vi "endsem.vi"() -> ()   [LabVIEW 2014]
uses:
  <vilib>/Analysis/NI_AALBase.lvlib
panel:
  out "XY Graph 2":cluster{dbl[], dbl[]}(graph)
  out "output cluster":cluster{dbl[], dbl[]}
  in  "standard deviation":dbl=1.0000000000000002 format="%0.2f"
  out "XY Graph":cdb[](graph)
  out "Array":i32[](array[numeric])
  in  "Numeric":i32
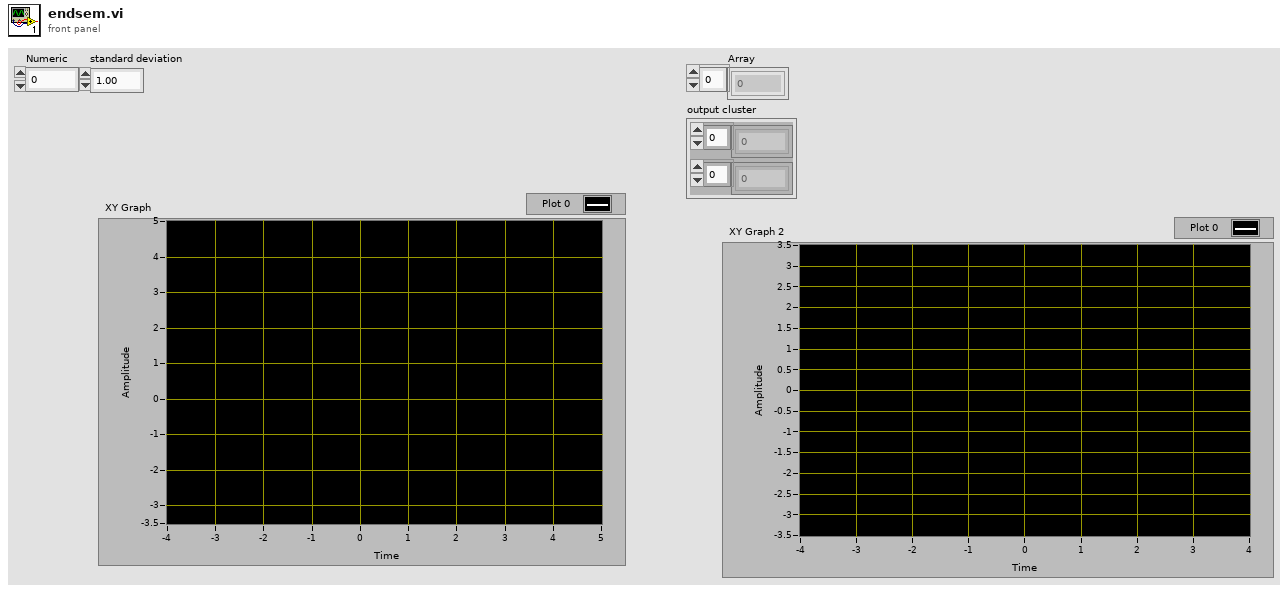
[diagram p1: front panel]
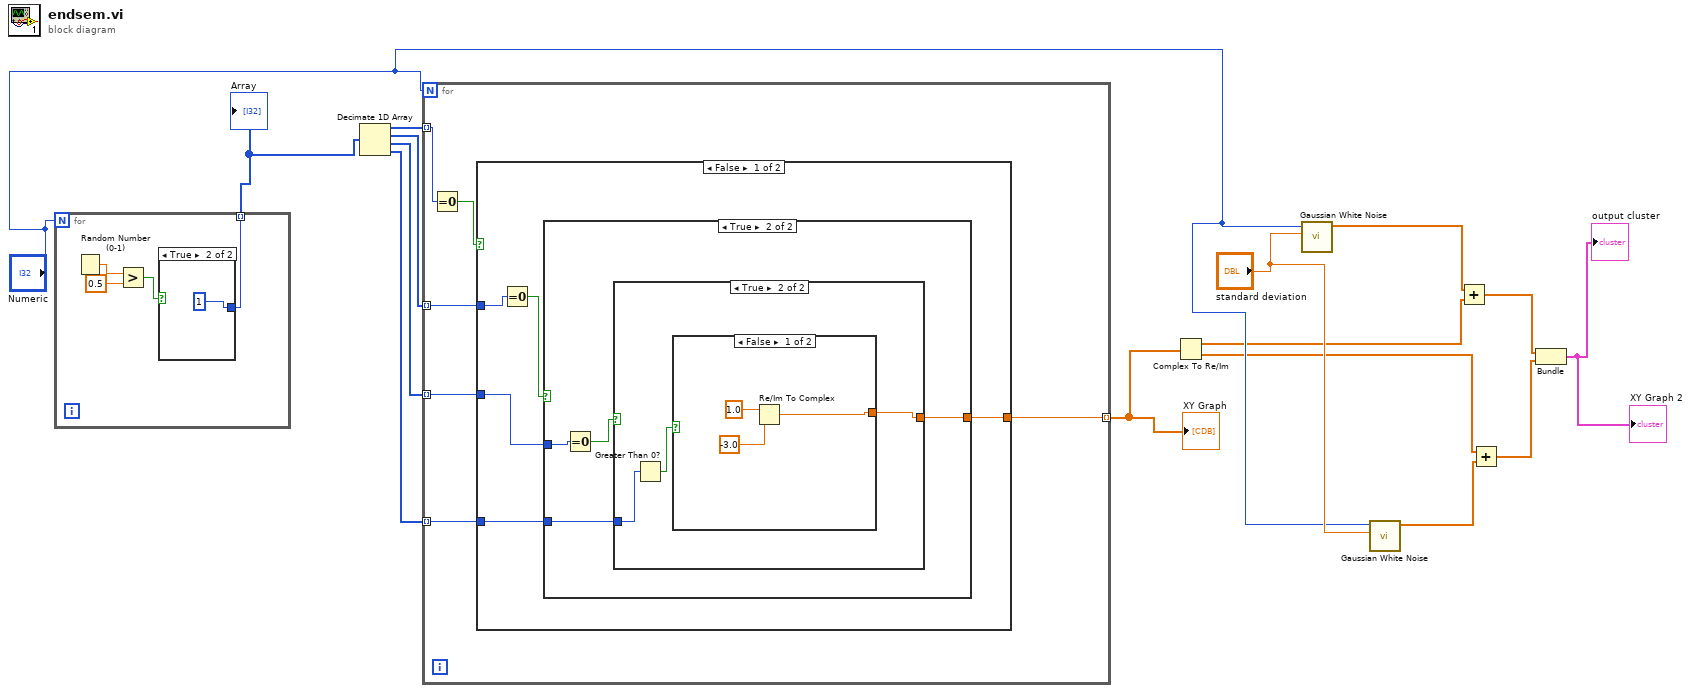
[diagram p0: block diagram]
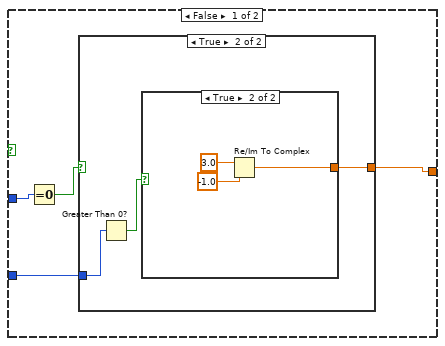
[diagram p2: hidden frame]
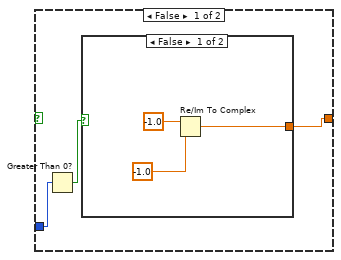
[diagram p3: hidden frame]
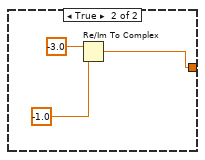
[diagram p4: hidden frame]
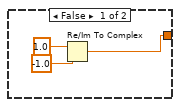
[diagram p5: hidden frame]
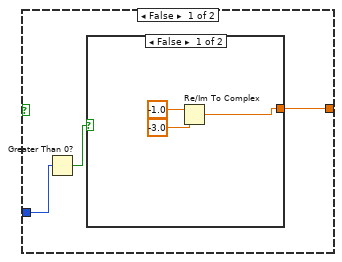
[diagram p6: hidden frame]
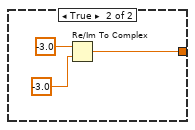
[diagram p7: hidden frame]
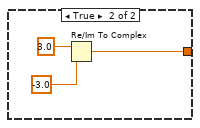
[diagram p8: hidden frame]
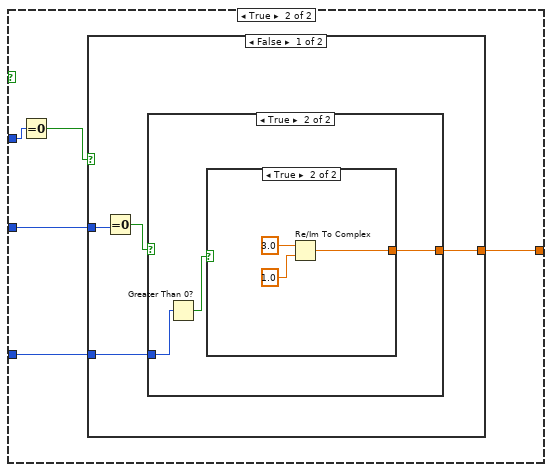
[diagram p9: hidden frame]
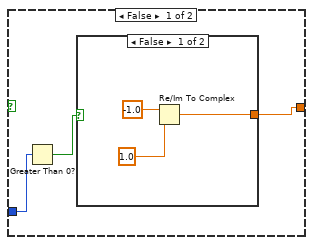
[diagram p10: hidden frame]
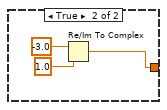
[diagram p11: hidden frame]
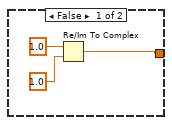
[diagram p12: hidden frame]
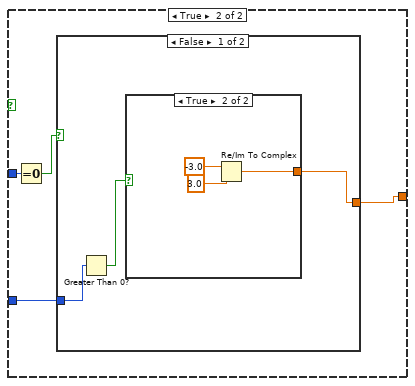
[diagram p13: hidden frame]
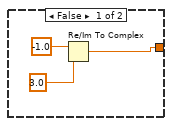
[diagram p14: hidden frame]
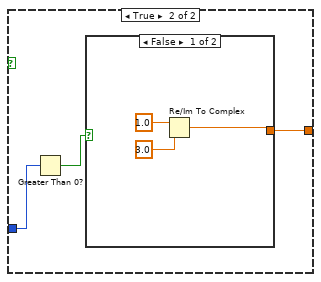
[diagram p15: hidden frame]
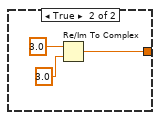
[diagram p16: hidden frame]
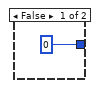
[diagram p17: hidden frame]
diagram:
  n1 = for {
    N: "Numeric" -> [_]
    tunnel: [w16] -> w15 mode=indexing
    n2 = Random Number (0-1)() -> (number: 0 to 1=w19:dbl)
    n3 = Greater?(x=w19, y=0.5) -> (0:w17:bool)
    n4 = case shown="True" w17 {
      tunnel: [0 1] -> w16
      frame False {
      }
      frame True {
      }
    }
  }
  "Array" <- w15
  n5 = Decimate 1D Array(w15) -> (w14:i32[], w13:i32[], w12:i32[], w11:i32[])
  n6 = for {
    N: "Numeric" -> [_]
    tunnel: w14 -> [w27] mode=indexing
    tunnel: w13 -> [w25] mode=indexing
    tunnel: w12 -> [w24] mode=indexing
    tunnel: w11 -> [w23] mode=indexing
    tunnel: [w22] -> w10 mode=indexing
    n7 = Equal To 0?(x=w27) -> (x = 0?=w26:bool)
    n8 = case shown="False" w26 {
      tunnel: w25 -> [w32 w81]
      tunnel: w24 -> [w30 w79]
      tunnel: w23 -> [w29 w78]
      tunnel: [w28 w77] -> w22
      frame False {
        n9 = Equal To 0?(x=w32) -> (x = 0?=w31:bool)
        n10 = case shown="True" w31 {
          tunnel: w30 -> [w36 w58]
          tunnel: w29 -> [w34 w56]
          tunnel: [w33 w55] -> w28
          frame False {
            n11 = Equal To 0?(x=w36) -> (x = 0?=w35:bool)
            n12 = case shown="True" w35 {
              tunnel: w34 -> [w39 w48]
              tunnel: [w37 w46] -> w33
              frame False {
                n13 = Greater Than 0?(x=w39) -> (x > 0?=w38:bool)
                n14 = case shown="False" w38 {
                  tunnel: [w40 w43] -> w37
                  frame False {
                    n15 = Re/Im To Complex(1:-1.0 ("y"), 2:-1.0 ("x")) -> (0:w40:cdb)
                  }
                  frame True {
                    n16 = Re/Im To Complex(1:-1.0 ("y"), 2:-3.0 ("x")) -> (0:w43:cdb)
                  }
                }
              }
              frame True {
                n17 = Greater Than 0?(x=w48) -> (x > 0?=w47:bool)
                n18 = case shown="True" w47 {
                  tunnel: [w49 w52] -> w46
                  frame False {
                    n19 = Re/Im To Complex(1:-1.0 ("y"), 2:1.0 ("x")) -> (0:w49:cdb)
                  }
                  frame True {
                    n20 = Re/Im To Complex(1:-1.0 ("y"), 2:3.0 ("x")) -> (0:w52:cdb)
                  }
                }
              }
            }
          }
          frame True {
            n21 = Equal To 0?(x=w58) -> (x = 0?=w57:bool)
            n22 = case shown="True" w57 {
              tunnel: w56 -> [w61 w70]
              tunnel: [w59 w68] -> w55
              frame False {
                n23 = Greater Than 0?(x=w61) -> (x > 0?=w60:bool)
                n24 = case shown="False" w60 {
                  tunnel: [w62 w65] -> w59
                  frame False {
                    n25 = Re/Im To Complex(1:-3.0 ("y"), 2:-1.0 ("x")) -> (0:w62:cdb)
                  }
                  frame True {
                    n26 = Re/Im To Complex(1:-3.0 ("x"), 2:-3.0 ("x")) -> (0:w65:cdb)
                  }
                }
              }
              frame True {
                n27 = Greater Than 0?(x=w70) -> (x > 0?=w69:bool)
                n28 = case shown="False" w69 {
                  tunnel: [w71 w74] -> w68
                  frame False {
                    n29 = Re/Im To Complex(1:-3.0 ("y"), 2:1.0 ("x")) -> (0:w71:cdb)
                  }
                  frame True {
                    n30 = Re/Im To Complex(1:-3.0 ("y"), 2:3.0 ("x")) -> (0:w74:cdb)
                  }
                }
              }
            }
          }
        }
      }
      frame True {
        n31 = Equal To 0?(x=w81) -> (x = 0?=w80:bool)
        n32 = case shown="False" w80 {
          tunnel: w79 -> [w85 w107]
          tunnel: w78 -> [w83 w105]
          tunnel: [w82 w104] -> w77
          frame False {
            n33 = Equal To 0?(x=w85) -> (x = 0?=w84:bool)
            n34 = case shown="True" w84 {
              tunnel: w83 -> [w88 w97]
              tunnel: [w86 w95] -> w82
              frame False {
                n35 = Greater Than 0?(x=w88) -> (x > 0?=w87:bool)
                n36 = case shown="False" w87 {
                  tunnel: [w89 w92] -> w86
                  frame False {
                    n37 = Re/Im To Complex(1:1.0 ("y"), 2:-1.0 ("x")) -> (0:w89:cdb)
                  }
                  frame True {
                    n38 = Re/Im To Complex(1:1.0 ("y"), 2:-3.0 ("x")) -> (0:w92:cdb)
                  }
                }
              }
              frame True {
                n39 = Greater Than 0?(x=w97) -> (x > 0?=w96:bool)
                n40 = case shown="True" w96 {
                  tunnel: [w98 w101] -> w95
                  frame False {
                    n41 = Re/Im To Complex(1:1.0 ("y"), 2:1.0 ("x")) -> (0:w98:cdb)
                  }
                  frame True {
                    n42 = Re/Im To Complex(1:1.0 ("y"), 2:3.0 ("x")) -> (0:w101:cdb)
                  }
                }
              }
            }
          }
          frame True {
            n43 = Equal To 0?(x=w107) -> (x = 0?=w106:bool)
            n44 = case shown="False" w106 {
              tunnel: w105 -> [w110 w119]
              tunnel: [w108 w117] -> w104
              frame False {
                n45 = Greater Than 0?(x=w110) -> (x > 0?=w109:bool)
                n46 = case shown="True" w109 {
                  tunnel: [w111 w114] -> w108
                  frame False {
                    n47 = Re/Im To Complex(1:3.0 ("y"), 2:-1.0 ("x")) -> (0:w111:cdb)
                  }
                  frame True {
                    n48 = Re/Im To Complex(1:3.0 ("y"), 2:-3.0 ("x")) -> (0:w114:cdb)
                  }
                }
              }
              frame True {
                n49 = Greater Than 0?(x=w119) -> (x > 0?=w118:bool)
                n50 = case shown="False" w118 {
                  tunnel: [w120 w123] -> w117
                  frame False {
                    n51 = Re/Im To Complex(1:3.0 ("y"), 2:1.0 ("x")) -> (0:w120:cdb)
                  }
                  frame True {
                    n52 = Re/Im To Complex(1:3.0 ("y"), 2:3.0 ("x")) -> (0:w123:cdb)
                  }
                }
              }
            }
          }
        }
      }
    }
  }
  "XY Graph" <- w10
  n53 = Complex To Re/Im(x + iy=w10) -> (x=w6:dbl[], y=w5:dbl[])
  n54 = call <vilib>:"Gaussian White Noise.vi"("standard deviation"="standard deviation", "samples"="Numeric") -> ("Gaussian noise pattern"=w7:dbl[])  [unwired: 8 in, 1 out]
  n55 = call <vilib>:"Gaussian White Noise.vi"("standard deviation"="standard deviation", "samples"="Numeric") -> ("Gaussian noise pattern"=w4:dbl[])  [unwired: 8 in, 1 out]
  n56 = Add(x=w7, y=w6) -> (x+y=w3:dbl[])
  n57 = Add(x=w5, y=w4) -> (x+y=w2:dbl[])
  n58 = Bundle(w3, w2) -> (→"output cluster" →"XY Graph 2":cluster{dbl[], dbl[]})  [unwired: 1 in]
